vi "tableNotification.vi"(8 "error in (no error)":errorcluster, 10 "Table in":refnum<vi>, 11 "reference in":refnum<class "Project Panels.lvclass">) -> (0 "error out":errorcluster, 3 "reference out":refnum<class "Project Panels.lvclass">)   [LabVIEW 2015, in "Project Panels.lvclass"]
uses:
  Project Panels.lvclass
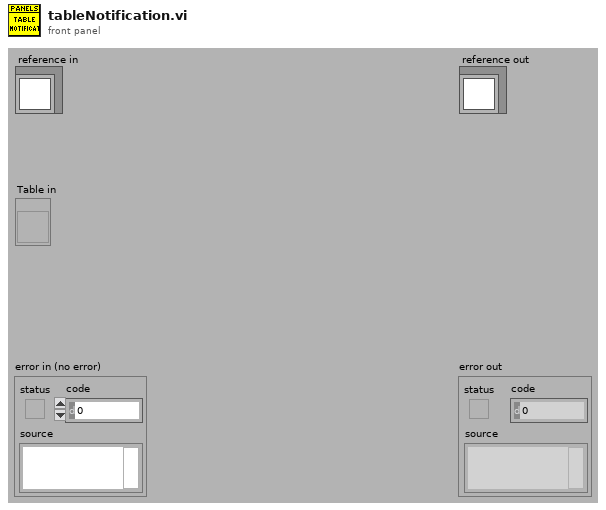
[diagram p1: front panel]
types:
  T1 = enum16{"User-specified Font", "Application Font", "System Font", "Dialog Font"}
  T2 = cluster{"Font Name:":string, "Size":i16, "Strikeout?":bool, "Italic?":bool, "Underline?":bool, "Outline?":bool, "Shadow?":bool, "Bold?":bool}
  T3 = typedef "Project Panels.lvclass/ObjectAttributesRef.ctl" = refnum<data-value>
  T4 = typedef "Project Panels.lvclass/ObjectAttributes.ctl" = cluster{"MyAttribute":dbl, "device_controller_ref":refnum<class "Devices Controller.lvclass">, "file_controller_ref":refnum<class "File Controller.lvclass">, "item_controller_ref":refnum<class "Items Controller.lvclass">, "item_tables":cluster{"checkIN":string[][], "checkOUT":string[][], "storage":string[][]}, "quickbook_table":cluster{"notes":string[][]}, "notification_controller_ref":refnum<class "Notification Controller.lvclass">, "partstracking_controller_ref":refnum<class "PartsTracking Controller.lvclass">, "product_tables":cluster{"k4b2":string[][], "fitmate":string[][], "RMR":string[][], "CPET":string[][], "BP":string[][], "PP":string[][], "k5":string[][], "bb-pft":string[][]}, "rowsColour":u32[], "low_resolution?":bool, "run_python?":bool}
  T5 = cluster{"left":i16, "top":i16, "right":i16, "bottom":i16}
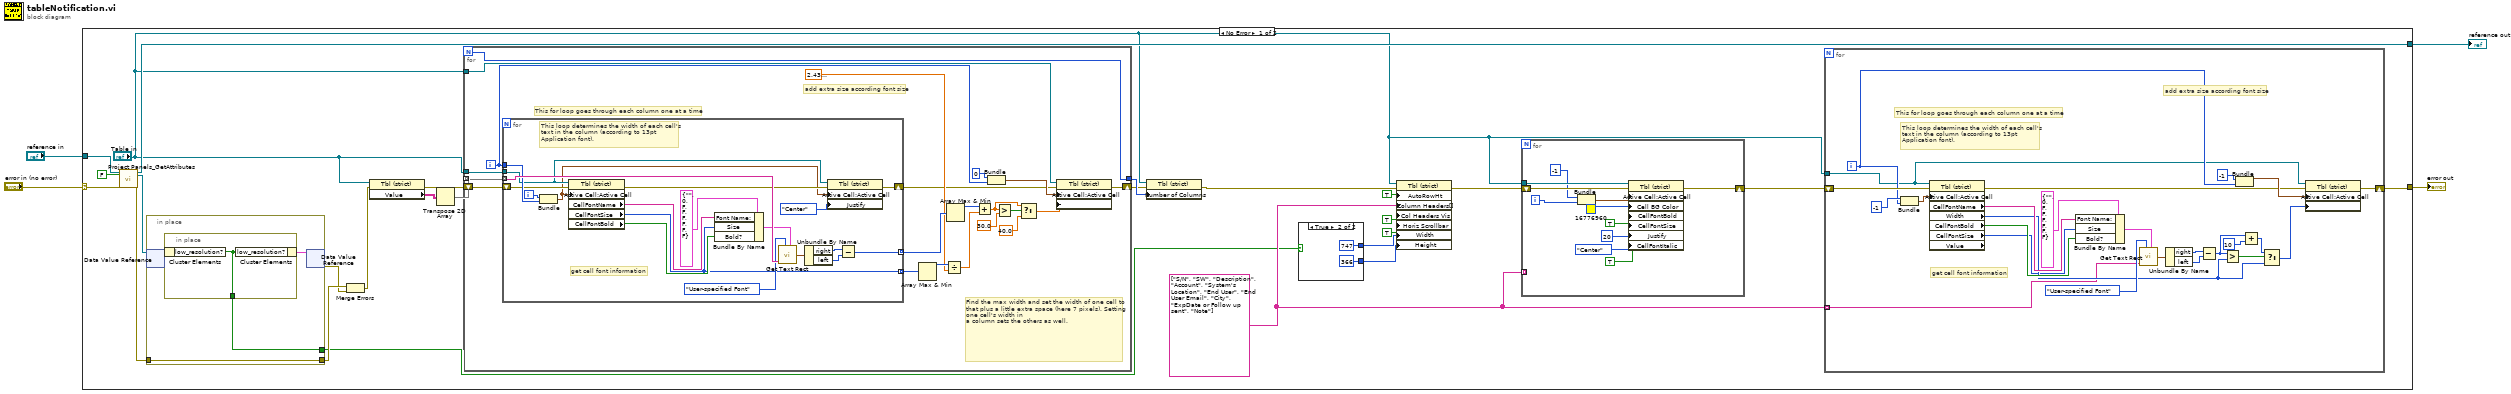
[diagram p0: block diagram]
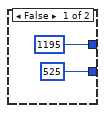
[diagram p2: hidden frame]
diagram:
  n1 = case shown="No Error" "error in (no error)" {
    selector: "error in (no error)" -> [w28 w117]
    tunnel: [w15 w117] -> w3
    tunnel: [w27 w116] -> w1
    tunnel: "reference in" -> [w30 w116]
    frame No Error {
      w11 = string[] ["S/N", "SW", "Description", "Account", "System's Location", "End User", "End User Email", "City", "ExpDate or Follow up sent", "Note"] ("Column Header Strings[]")
      n2 = call "Project Panels_GetAttributes.vi"("reference in"=w30, "return data? (T)"=FALSE, "error in (no error)"=w28) -> ("reference out"=w27:refnum<class "Project Panels.lvclass">, "attributes ref"=w7:T3, "error out"=w8:errorcluster)  [unwired: 13 in, 1 out]
      n3 = in-place {
        in-place-border: w8 -> [w32]
        in-place-border: [w32] -> w10
        in-place-border: [w31] -> w5
        n4 = in-place-dvr #1(w7) -> (w33:T4)  [unwired: 1 out]
        n5 = in-place {
          in-place-border: [w35] -> w31
          n6 = in-place-cluster #2(w33) -> ("low_resolution?"=w35:bool)
          n7 = in-place-cluster #2("low_resolution?"=w35) -> (w34:T4)
        }
        n8 = in-place-dvr #1(w34) -> (w9:errorcluster)  [unwired: 1 out]
      }
      n9 = Merge Errors(w10, w9) -> (w6:errorcluster)
      n10 = property on="Property Node" class="Tbl (strict)"(reference="Table in", error in=w6) -> (error out=w22:errorcluster, "Value"=w23:string[][])  [unwired: 1 out]
      n11 = Transpose 2D Array(2D array=w23) -> (transposed array=w24:string[][])
      n12 = for {
        N -> [w85]
        tunnel: w24 -> [w96] mode=indexing
        tunnel: [w85] -> w26
        tunnel: "Table in" -> [w84]
        tunnel: "Table in" -> [w83]
        shift-right: [w86] -> w25
        shift-left: w22 -> [w82]
        i -> [w92]
        # "add extra size according font size"
        # "Find the max width and set the width of one cell to that plus a little extra space (here 7 pixels). Setting one cell's width in\na column sets the others as well."
        # "This for loop goes through each column one at a time"
        n13 = for {
          tunnel: w96 -> [w115] mode=indexing
          tunnel: [w111] -> w95 mode=indexing
          tunnel: w92 -> [w106]
          tunnel: [w103] -> w90 mode=indexing
          tunnel: w84 -> [w98]
          shift-right: [w100] -> w81
          shift-left: w82 -> [w102]
          i -> [w105]
          # "get cell font information"
          # "This loop determines the width of each cell's\ntext in the column (according to 13pt\nApplication font)."
          n14 = Bundle(w105, w106) -> (w97:cluster{i32, i32})  [unwired: 1 in]
          n15 = property on="Property Node" class="Tbl (strict)"(reference=w98, error in=w102, "Active Cell:Active Cell"=w97) -> (error out=w101:errorcluster, "CellFontName"=w110:string, "CellFontSize"=w103:u32, "CellFontBold"=w109:bool)  [unwired: 1 out]
          n16 = Bundle By Name(cluster=T2 {"Font Name:"="", "Size"=0, "Strikeout?"=FALSE, "Italic?"=FALSE, "Underline?"=FALSE, "Outline?"=FALSE, "Shadow?"=FALSE, "Bold?"=FALSE} ("[user-specified font]"), "Font Name:"=w110, "Size"=w103, "Bold?"=w109) -> (w107:T2)
          n17 = call <vilib>:"Get Text Rect.vi"("desired font(Application)"=T1."User-specified Font", "text"=w115, "[user-specified font]"=w107) -> ("rect"=w114:T5)  [unwired: 6 in]
          n18 = Unbundle By Name(w114) -> ("right"=w113:i16, "left"=w112:i16)
          n19 = property on="Property Node" class="Tbl (strict)"(reference=w98, error in=w101, "Active Cell:Active Cell"=w97, "Justify"=enum16{"Left", "Center", "Right"}."Center" ("Active Cell:Cell Justification")) -> (error out=w100:errorcluster)  [unwired: 1 out]
          n20 = Subtract(x=w113, y=w112) -> (x-y=w111:i16)
        }
        n21 = Array Max & Min(array=w90) -> (max value=w89:u32)  [unwired: 3 out]
        n22 = Divide(x=w89, y=sgl 2.43) -> (x/y=w87:sgl)
        n23 = Array Max & Min(array=w95) -> (max value=w91:i16)  [unwired: 3 out]
        n24 = Add(x=w91, y=w87) -> (x+y=w76:sgl)
        n25 = Bundle(0, w92) -> (w93:cluster{i32, i32})  [unwired: 1 in]
        n26 = Greater?(x=w76, y=sgl 30.0) -> (0:w79:bool)
        n27 = Select(t=w76, s=w79, f=sgl 40.0 ("y")) -> (s? t:f=w78:sgl)
        n28 = property on="Property Node" class="Tbl (strict)"(reference=w83, error in=w81, "Active Cell:Active Cell"=w93, "Active Cell:Cell Size:Width"=w78) -> (error out=w86:errorcluster)  [unwired: 1 out]
      }
      n29 = property on="Property Node" class="Tbl (strict)"(reference="Table in", error in=w25, "Number of Columns"=w26) -> (error out=w16:errorcluster)  [unwired: 1 out]
      n30 = case shown="True" w5 {
        tunnel: [u32 1195 ("Size:Width") u32 747 ("Size:Width")] -> w18
        tunnel: [u32 525 ("Size:Width") u32 366 ("Size:Width")] -> w17
        frame False {
        }
        frame True {
        }
      }
      n31 = property on="Property Node" class="Tbl (strict)"(reference="Table in", error in=w16, "AutoRowHt"=TRUE ("Autosizing Row Height"), "Column Headers[]"=w11, "Col Headers Vis"=TRUE ("Visible Items:Column Headers Visible"), "Horiz Scrollbar"=TRUE ("Visible Items:Horizontal Scrollbar Visible"), "Width"=w18, "Height"=w17) -> (error out=w14:errorcluster)  [unwired: 1 out]
      n32 = for {
        tunnel: "Table in" -> [w48]
        tunnel: w11 -> [_] mode=indexing
        shift-right: [w49] -> w13
        shift-left: w14 -> [w50]
        i -> [w46]
        n33 = Bundle("index"=-1, w46) -> (w47:cluster{"index":i32, i32})  [unwired: 1 in]
        n34 = property on="Property Node" class="Tbl (strict)"(reference=w48, error in=w50, "Active Cell:Active Cell"=w47, "Cell BG Color"=u32 16776960, "CellFontBold"=TRUE ("Active Cell:Cell Font:Bold"), "CellFontSize"=u32 20 ("Active Cell:Cell Font:Size"), "Justify"=enum16{"Left", "Center", "Right"}."Center" ("Active Cell:Cell Justification"), "CellFontItalic"=TRUE ("Active Cell:Cell Font:Italic")) -> (error out=w49:errorcluster)  [unwired: 1 out]
      }
      n35 = for {
        tunnel: "Table in" -> [w54]
        shift-right: [w73] -> w15
        shift-left: w13 -> [w72]
        tunnel: w11 -> [w52] mode=indexing
        i -> [w61]
        # "get cell font information"
        # "This loop determines the width of each cell's\ntext in the column (according to 13pt\nApplication font)."
        # "add extra size according font size"
        # "This for loop goes through each column one at a time"
        n36 = Bundle("index"=-1, w61) -> (w60:cluster{"index":i32, i32})  [unwired: 1 in]
        n37 = property on="Property Node" class="Tbl (strict)" props=["Active Cell:Active Cell", "CellFontName", "Width", "CellFontBold", "CellFontSize", "Value"](reference=w54, error in=w72, "Active Cell:Active Cell"=w60) -> (error out=w51:errorcluster, "CellFontName"=w67:string, "Width"=w55:u32, "CellFontBold"=w66:bool, "CellFontSize"=w53:u32)  [unwired: 2 out]
        n38 = Bundle By Name(cluster=T2 {"Font Name:"="", "Size"=0, "Strikeout?"=FALSE, "Italic?"=FALSE, "Underline?"=FALSE, "Outline?"=FALSE, "Shadow?"=FALSE, "Bold?"=FALSE} ("[user-specified font]"), "Font Name:"=w67, "Size"=w53, "Bold?"=w66) -> (w64:T2)
        n39 = call <vilib>:"Get Text Rect.vi"("desired font(Application)"=T1."User-specified Font", "text"=w52, "[user-specified font]"=w64) -> ("rect"=w70:T5)  [unwired: 6 in]
        n40 = Unbundle By Name(w70) -> ("right"=w69:i16, "left"=w68:i16)
        n41 = Subtract(x=w69, y=w68) -> (x-y=w58:i16)
        n42 = Greater?(x=w58, y=w55) -> (0:w59:bool)
        n43 = Bundle(-1, w61) -> (w74:cluster{i32, i32})  [unwired: 1 in]
        n44 = Add(x=w58, y=i16 10) -> (x+y=w56:i16)
        n45 = Select(t=w56, s=w59, f=w55) -> (s? t:f=w71:u32)
        n46 = property on="Property Node" class="Tbl (strict)"(reference=w54, error in=w51, "Active Cell:Active Cell"=w74, "Active Cell:Cell Size:Width"=w71) -> (error out=w73:errorcluster)  [unwired: 1 out]
      }
    }
    frame Error {
    }
  }
  "error out" <- w3
  "reference out" <- w1
